vi "configure.vi"() -> (0 "show samples per acquisition":dbl, 2 "show sampling rate (samples/sec)":dbl)   [LabVIEW 2014]
panel:
  in  "OK Button":bool
  in  "samples per acquisition":dbl=10000.0
  in  "sampling rate (samples/sec)":dbl=1000.0
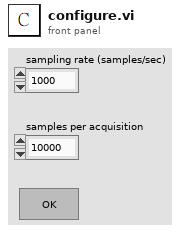
[diagram p1: front panel]
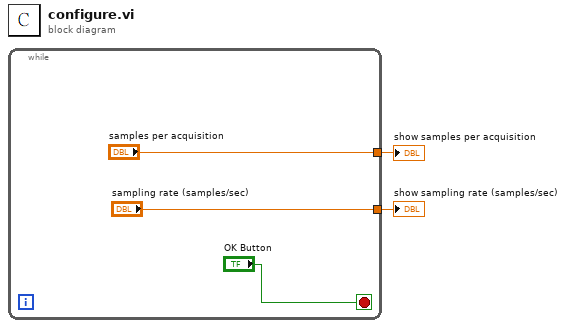
[diagram p0: block diagram]
diagram:
  n1 = while {
    tunnel: ["samples per acquisition"] -> w2
    tunnel: ["sampling rate (samples/sec)"] -> w1
    stop <- "OK Button" stop-if-true
  }
  "show samples per acquisition" <- w2
  "show sampling rate (samples/sec)" <- w1
